vi "Close.vi"(8 "error in (no error)":errorcluster, 11 "RTL-SDR in":refnum<class "Session.lvclass">) -> (0 "error out":errorcluster, 3 "Device":refnum<class "Device.lvclass">)   [LabVIEW 2020, in "RTL-SDR.lvlib" / "Session.lvclass"]
uses:
  Session.lvclass
  C:/dev/IlluminatedG/lv-rtl-sdr/lib/librtlsdr.dll
  Device/Device.lvclass
panel:
  out "return type":i32
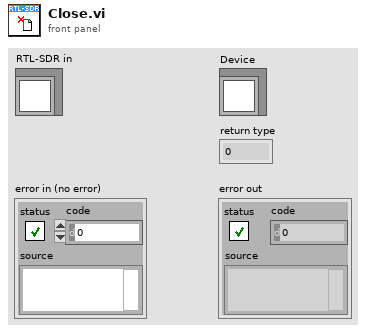
[diagram p1: front panel]
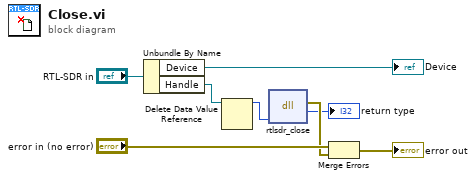
[diagram p0: block diagram]
diagram:
  n1 = Unbundle By Name("RTL-SDR in") -> ("Device"=→"Device":refnum<class "Device.lvclass">, "Handle"=w2:refnum<data-value>)
  n2 = Delete Data Value Reference(data value reference=w2) -> (data value=w1:u64)  [unwired: 1 in, 1 out]
  n3 = dll-call lib="C:/dev/IlluminatedG/lv-rtl-sdr/lib/librtlsdr.dll" fn="rtlsdr_close"("dev"=w1) -> (error out=w5:errorcluster, "return type"=→"return type":i32)  [unwired: 4 in, 1 out]
  n4 = Merge Errors("error in (no error)", w5) -> (→"error out":errorcluster)
